vi "Bury.vi"(8 "Error In":errorcluster) -> (0 "Error Out":errorcluster)   [LabVIEW 2018, in "Tests.lvlib" / "Toolkit.lvlib" / "Integration.lvlib"]
uses:
  Integration.lvlib
  src/Toolkit/Toolkit.lvlib
  <vilib>/addons/_JKI Toolkits/Caraya/classes/Test/Test.lvclass
  <vilib>/addons/_JKI Toolkits/Caraya/classes/Assert/Assert.lvclass
  Tests.lvlib
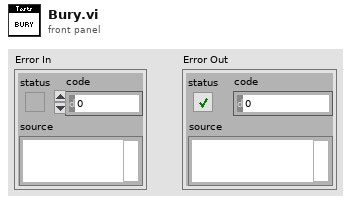
[diagram p1: front panel]
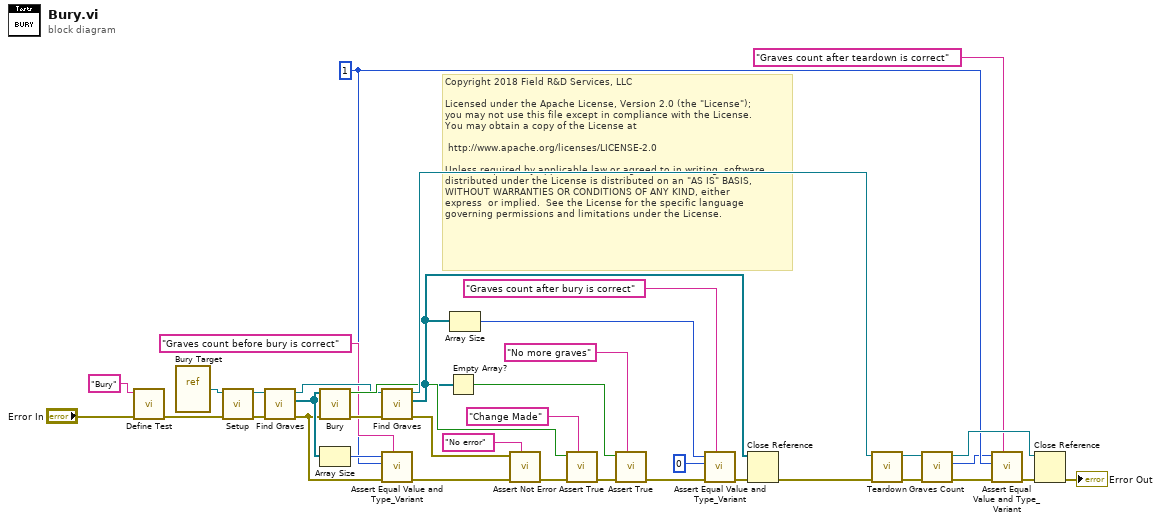
[diagram p0: block diagram]
diagram:
  w5 = 1 ("size(s)")
  # "Copyright 2018 Field R&D Services, LLC\n\nLicensed under the Apache License, Version 2.0 (the \"License\");\nyou may not use this file except in compliance with the License.\nYou may obtain a copy of the License at\n\n\thttp://www.apache.org/licenses/LICENSE-2.0\n\nUnless required by applicable law or agreed to in writing, software\ndistributed under the License is distributed on an \"AS IS\" BASIS,\nWITHOUT WARRANTIES OR CONDITIONS OF ANY KIND, either \nexpress  or implied.  See the License for the specific language \ngoverning permissions and limitations under the License."
  n1 = call <vilib>:"Define Test.vi"("error in (no error)"="Error In", "Label (VI Title)"="Bury") -> ("error out"=w23:errorcluster)  [unwired: 9 in]
  n2 = vi-ref "Bury Target.vi"() -> (w22:refnum<vi>)
  n3 = call "Setup.vi"("Error In"=w23, "VI In"=w22) -> ("Error Out"=w1:errorcluster, "VI Out"=w2:refnum<vi>)  [unwired: 8 in]
  n4 = call "Find Graves.vi"("Error In"=w1, "VI In"=w2) -> ("Error Out"=w20:errorcluster, "Graves"=w21:refnum<vi>[], "VI Out"=w26:refnum<vi>)  [unwired: 7 in]
  n5 = call "Bury.vi"("Error In"=w20, "Graves"=w21) -> ("Error Out"=w38:errorcluster, "Change Made?"=w28:bool)  [unwired: 8 in]
  n6 = Array Size(array=w21) -> (size(s)=w18:i32)
  n7 = call "Find Graves.vi"("Error In"=w38, "VI In"=w26) -> ("Error Out"=w33:errorcluster, "Graves"=w14:refnum<vi>[], "VI Out"=w31:refnum<vi>)  [unwired: 7 in]
  n8 = call <vilib>:"Assert Equal Value and Type_Variant.vi"("Label"="Graves count before bury is correct", "error in (no error)"=w20, "Y"=w5, "X"=w18) -> ("error out"=w19:errorcluster)  [unwired: 7 in]
  n9 = Empty Array?(array=w14) -> (empty?=w25:bool)
  n10 = Array Size(array=w14) -> (size(s)=w13:i32)
  n11 = call <vilib>:"Assert Not Error.vi"("Label"="No error", "error in (no error)"=w19, "Not Error?"=w33) -> ("error out"=w35:errorcluster)  [unwired: 8 in]
  n12 = call <vilib>:"Assert True.vi"("Label"="Change Made", "error in (no error)"=w35, "True?"=w28) -> ("error out"=w29:errorcluster)  [unwired: 8 in]
  n13 = call <vilib>:"Assert True.vi"("Label"="No more graves", "error in (no error)"=w29, "True?"=w25) -> ("error out"=w16:errorcluster)  [unwired: 8 in]
  n14 = call <vilib>:"Assert Equal Value and Type_Variant.vi"("Label"="Graves count after bury is correct", "error in (no error)"=w16, "Y"=0 ("size(s)"), "X"=w13) -> ("error out"=w15:errorcluster)  [unwired: 7 in]
  n15 = Close Reference(reference=w14, error in (no error)=w15) -> (error out=w24:errorcluster)
  n16 = call "Teardown.vi"("Error In"=w24, "VI In"=w31) -> ("Error Out"=w8:errorcluster, "VI Out"=w10:refnum<vi>)  [unwired: 8 in]
  n17 = call "Graves Count.vi"("Error In"=w8, "Test Target In"=w10) -> ("Error Out"=w3:errorcluster, "Graves Count"=w4:i32, "Test Target Out"=w9:refnum<vi>)  [unwired: 7 in]
  n18 = call <vilib>:"Assert Equal Value and Type_Variant.vi"("Label"="Graves count after teardown is correct", "error in (no error)"=w3, "Y"=w5, "X"=w4) -> ("error out"=w7:errorcluster)  [unwired: 7 in]
  n19 = Close Reference(reference=w9, error in (no error)=w7) -> (error out=→"Error Out":errorcluster)
